vi "getActionPanelPath.vi"(8 "error in (no error)":errorcluster, 11 "ActionPanel in":refnum<class "ActionPanel.lvclass">) -> (0 "error out":errorcluster, 2 "frontPanelPath":path, 3 "ActionPanel out":refnum<class "ActionPanel.lvclass">)   [LabVIEW 2011, in "Views.lvlib" / "ScriptEditor.lvlib" / "ActionPanel.lvclass"]
uses:
  ActionPanel.lvclass
  Tools/Filing/FileSystem/FileSystem.lvclass
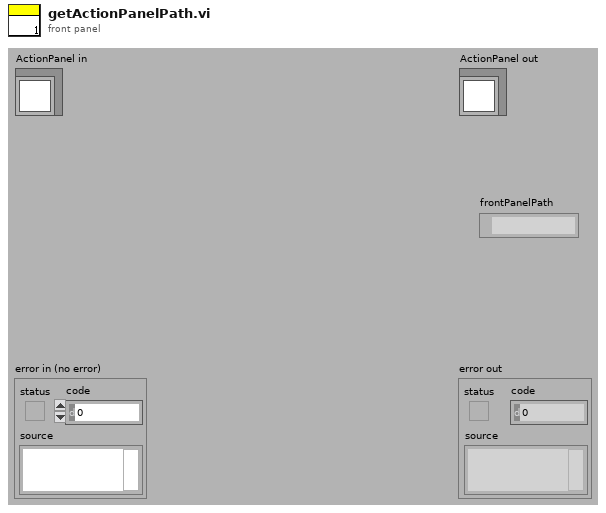
[diagram p1: front panel]
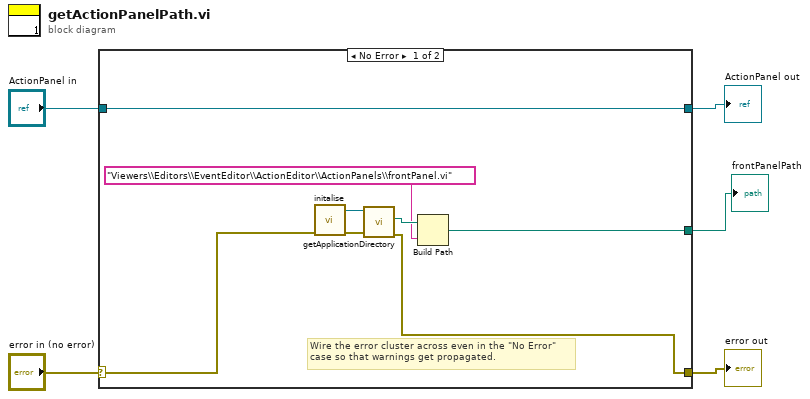
[diagram p0: block diagram]
diagram:
  n1 = case shown="No Error" "error in (no error)" {
    selector: "error in (no error)" -> [w6 w15]
    tunnel: [w7 w15] -> w4
    tunnel: [w13 w14] -> w2
    tunnel: "ActionPanel in" -> [w13 w14]
    tunnel: [w8 _] -> w1
    frame No Error {
      # "Wire the error cluster across even in the \"No Error\"\ncase so that warnings get propagated."
      n2 = call "initalise.vi"("error in (no error)"=w6) -> ("error out"=w12:errorcluster, "FileSystem out"=w11:refnum<class "FileSystem.lvclass">)  [unwired: 9 in]
      n3 = call-dynamic "getApplicationDirectory.vi"("error in (no error)"=w12, "FileSystem.lvclass in"=w11) -> ("error out"=w7:errorcluster, "ApplicationDirectory"=w10:path)  [unwired: 7 in, 1 out]
      n4 = Build Path(base path=w10, name or relative path="Viewers\\Editors\\EventEditor\\ActionEditor\\ActionPanels\\frontPanel.vi") -> (appended path=w8:path)
    }
    frame Error {
    }
  }
  "error out" <- w4
  "ActionPanel out" <- w2
  "frontPanelPath" <- w1
